vi "CRC16.vi"(11 "buf":string) -> (1 "CRCLo":u8 format="%x", 2 "CRCHi":u8 format="%x", 3 "CRC":u16 format="%x")   [LabVIEW 2016, in "数据传输系统-04.lvlib"]
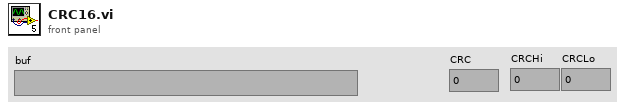
[diagram p1: front panel]
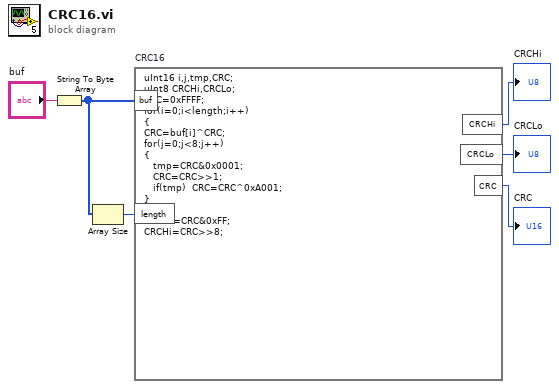
[diagram p0: block diagram]
diagram:
  n1 = String To Byte Array(string="buf") -> (unsigned byte array=w1:u8[])
  n2 = Array Size(array=w1) -> (size(s)=w4:i32)
  n3 = formula code="uInt16 i,j,tmp,CRC;\nuInt8 CRCHi,CRCLo;\nCRC=0xFFFF; \nfor(i=0;i<length;i++)\n{ \nCRC=buf[i]^CRC;  \nfor(j=0;j<8;j++)   \n{   \n   tmp=CRC&0x0001;    \n   CRC=CRC>>1;  \n   if(tmp)  CRC=CRC^0xA001;  \n} \n} \nCRCLo=CRC&0xFF;\nCRCHi=CRC>>8;" "CRC16"("buf"=w1, "length"=w4) -> ("CRCHi"=→"CRCHi":u8, "CRCLo"=→"CRCLo":u8, "CRC"=→"CRC":u16)
